vi "Joystick Analyze.vi"(2 "Joystick Name":T2) -> (3 "DriveSlow":bool, 4 "Stabilize Gain":dbl, 5 "ResetGyro":bool, 6 "x":dbl, 7 "y":dbl, 9 "Stabilize":bool, 10 "JackControl":T1)   [LabVIEW 2011]
uses:
  <vilib>/Rock Robotics/WPI/Joystick/WPI_JoystickDevRef.ctl
  <vilib>/Rock Robotics/WPI/Joystick/WPI_JoystickDeviceEnum.ctl
  <vilib>/Rock Robotics/WPI/Relay/WPI_RelayValue.ctl
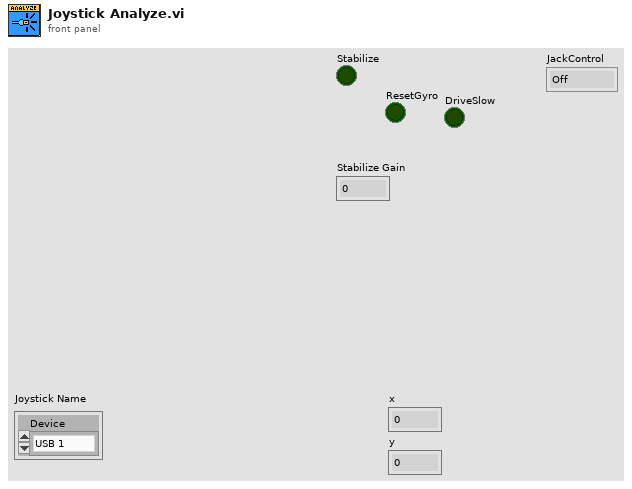
[diagram p1: front panel]
types:
  T1 = typedef "WPI_RelayValue.ctl" = enum16{"Off", "On", "Forward", "Reverse"}
  T2 = typedef "WPI_JoystickDevRef.ctl" = cluster{"Device":T3}
  T3 = typedef "WPI_JoystickDeviceEnum.ctl" = enum16{"USB 1", "USB 2", "USB 3", "USB 4", "Kinect 1", "Kinect 2"}
  T4 = typedef "WPI_JoystickButtonState.ctl" = cluster{"Button 1":bool, "Button 2":bool, "Button 3":bool, "Button 4":bool, "Button 5":bool, "Button 6":bool, "Button 7":bool, "Button 8":bool, "Button 9":bool, "Button 10":bool, "Button 11":bool, "Button 12":bool}
  T5 = cluster{"axis 1 (x)":dbl, "axis 2 (y)":dbl, "axis 3 (throttle)":dbl, "axis 4":dbl, "axis 5":dbl, "axis 6":dbl}
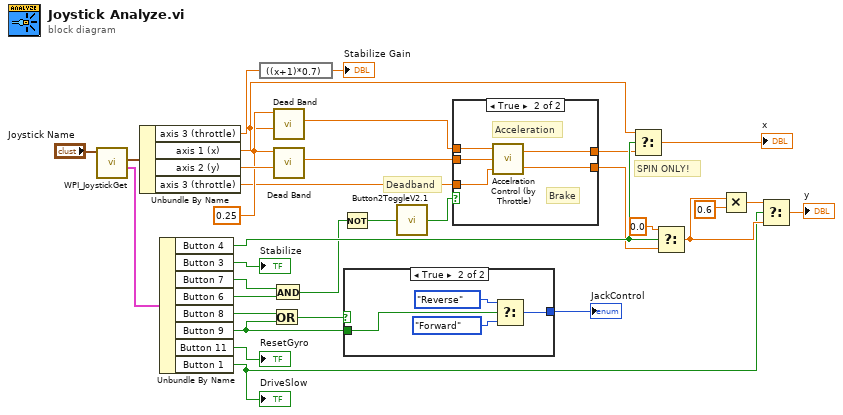
[diagram p0: block diagram]
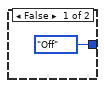
[diagram p2: hidden frame]
diagram:
  w28 = 0.25 ("Dead Band")
  # "Deadband"
  # "SPIN ONLY!"
  n1 = call <vilib>:"WPI_JoystickGet.vi"("JoystickDevRef"="Joystick Name") -> ("Buttons"=w31:T4, "Axes"=w32:T5)  [unwired: 1 in, 4 out]
  n2 = Unbundle By Name(w32) -> ("axis 3 (throttle)"=w13:dbl, "axis 1 (x)"=w18:dbl, "axis 2 (y)"=w29:dbl, "axis 3 (throttle)"=w21:dbl)
  n3 = Unbundle By Name(w31) -> ("Button 4"=w27:bool, "Button 3"=→"Stabilize":bool, "Button 7"=w16:bool, "Button 6"=w15:bool, "Button 8"=w3:bool, "Button 9"=w2:bool, "Button 11"=→"ResetGyro":bool, "Button 1"=w5:bool)
  "DriveSlow" <- w5
  n4 = expression code="((x+1)*0.7)"(w13) -> (→"Stabilize Gain":dbl)
  n5 = Or(x=w3, y=w2) -> (x .or. y?=w4:bool)
  n6 = And(x=w16, y=w15) -> (x .and. y?=w12:bool)
  n7 = call "Dead Band.vi"("Axis In"=w18, "Dead Band"=w28) -> ("Axis Out"=w23:dbl)  [unwired: 9 in]
  n8 = call "Dead Band.vi"("Axis In"=w29, "Dead Band"=w28) -> ("Axis Out"=w22:dbl)  [unwired: 9 in]
  n9 = Not(x=w12) -> (.not. x?=w7:bool)
  n10 = case shown="True" w4 {
    tunnel: [WPI_RelayValue."Off" ("RelayValue") w35] -> w1
    tunnel: w2 -> [_ w34]
    frame False {
    }
    frame True {
      n11 = Select(t=WPI_RelayValue."Reverse" ("RelayValue"), s=w34, f=WPI_RelayValue."Forward" ("RelayValue")) -> (s? t:f=w35:T1)
    }
  }
  "JackControl" <- w1
  n12 = call "Button2ToggleV2.1.vi"("a"=w7) -> ("Result(clone)"=w6:bool)
  n13 = case shown="True" w6 {
    tunnel: w23 -> [w39 w41]
    tunnel: w22 -> [w38 w42]
    tunnel: w21 -> [_ w40]
    tunnel: [w39 w44] -> w20
    tunnel: [w38 w43] -> w19
    frame False {
    }
    frame True {
      # "Brake"
      # "Acceleration"
      n14 = call "Accelration Control (by Throttle).vi"("acc"=w40, "Yinput"=w42, "Xinput"=w41) -> ("Youtput"=w43:dbl, "Xoutput"=w44:dbl)
    }
  }
  n15 = Select(t=w18, s=w27, f=w20) -> (s? t:f=→"x":dbl)
  n16 = Select(t=0.0, s=w27, f=w19) -> (s? t:f=w10:dbl)
  n17 = Multiply(x=w10, y=0.6) -> (x*y=w9:dbl)
  n18 = Select(t=w9, s=w5, f=w10) -> (s? t:f=→"y":dbl)
